vi "例3.4.vi"() -> ()   [LabVIEW 2017]
panel:
  out "子字符串":string
  out "数值":dbl
  in  "输入字符串":string
  in  "偏移量(0) 2":i32
  in  "长度（剩余）":i32
  in  "偏移量(0)":i32
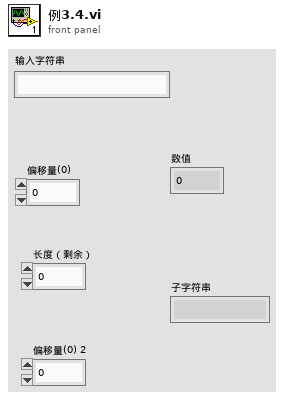
[diagram p1: front panel]
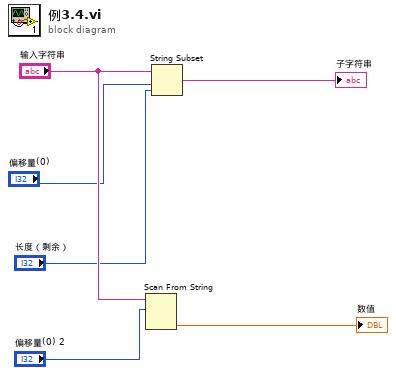
[diagram p0: block diagram]
diagram:
  n1 = Scan From String(input string="输入字符串", initial scan location="偏移量(0) 2") -> (output 1=→"数值":dbl)  [unwired: 3 in, 3 out]
  n2 = String Subset(string="输入字符串", offset (0)="偏移量(0)", length (rest)="长度（剩余）") -> (substring=→"子字符串":string)
